vi "Stop Core.vi"(10 "final error code":i32, 11 "ServerUI in":refnum<class "ServerUI.lvclass">) -> (3 "ServerUI out":refnum<class "ServerUI.lvclass">)   [LabVIEW 2018, in "ServerUI.lvlib" / "ServerUI.lvclass"]
doc: "(<B>Filename</B>: Actor Framework.lvlib:Actor.lvclass:Stop Core.vi)\n\nDefines what the actor does before it stops. Use the <B>final error code</B> input to determine whether the actor shut down in response to an error.\n\nBy default, this method passes the Stop message along to all auto-stop nested actors. A descendant class may override this method to define additional behavior, such as shutting down any processes the actor initiated in its override of the Actor Core method."
uses:
  ServerUI.lvclass
  ServerUI.lvclass/ServerUI.ctl
  TCP_Server/TCP_Server/TCP_Server.lvclass
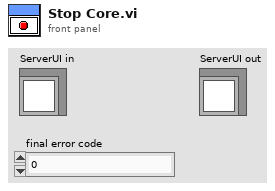
[diagram p1: front panel]
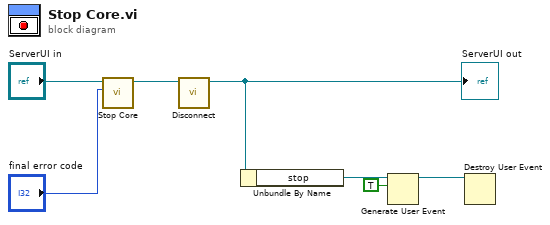
[diagram p0: block diagram]
diagram:
  n1 = call-parent "Stop Core.vi"("final error code"="final error code", "Actor in"="ServerUI in") -> ("Actor out"=w2:refnum<class "ServerUI.lvclass">)  [unwired: 9 in]
  n2 = call-dynamic "Disconnect.vi"("TCP_Client in"=w2) -> ("TCP_Client out"=w1:refnum<class "ServerUI.lvclass">)  [unwired: 9 in, 1 out]
  "ServerUI out" <- w1
  n3 = Unbundle By Name(w1) -> ("stop"=w5:refnum<user-event>)
  n4 = Generate User Event(user event=w5, event data cluster=TRUE ("event data")) -> (user event out=w3:refnum<user-event>)  [unwired: 2 in, 1 out]
  n5 = Destroy User Event(user event=w3) -> ()  [unwired: 1 in, 1 out]
